vi "labview_data Writer Example.vi"() -> ()   [LabVIEW 2024]
uses:
  <vilib>/RTI DDS Toolkit/Types/RTI DDS Advanced Writer Configuration.ctl
  <vilib>/RTI DDS Toolkit/Library/LVDDS_library.lvlib
panel:
  in  "Sample":T1
  in  "Sample Type":T1
  in  "Advanced Writer Configuration":T2
  in  "error in (no error)":errorcluster
  in  "Stop Writing":bool
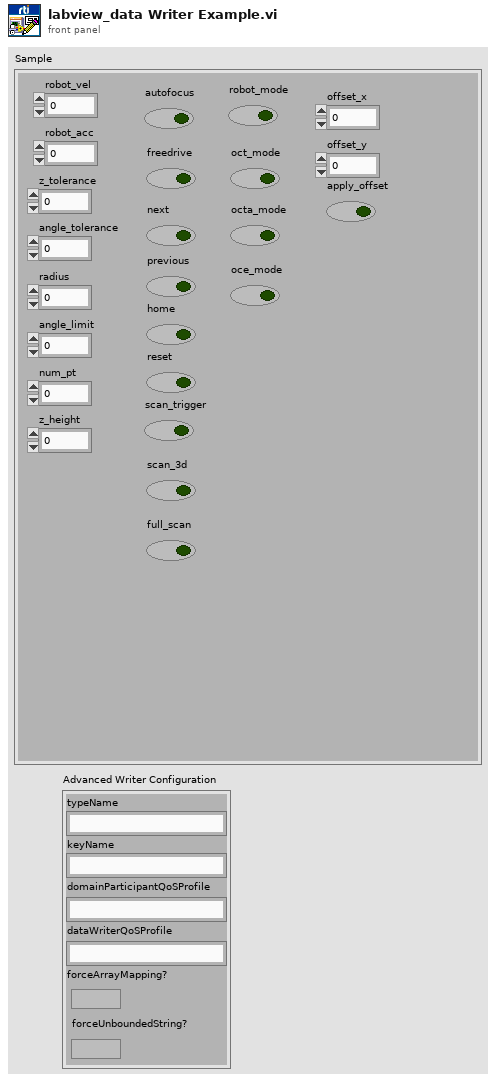
[diagram p1: front panel]
types:
  T1 = cluster{"robot_vel":dbl, "robot_acc":dbl, "z_tolerance":dbl, "angle_tolerance":dbl, "radius":dbl, "angle_limit":dbl, "num_pt":i32, "z_height":dbl, "autofocus":bool, "freedrive":bool, "next":bool, "previous":bool, "home":bool, "reset":bool, "scan_trigger":bool, "scan_3d":bool, "full_scan":bool, "robot_mode":bool, "oct_mode":bool, "octa_mode":bool, "oce_mode":bool, "offset_x":dbl, "offset_y":dbl, "apply_offset":bool}
  T2 = typedef "LVDDS_library.lvlib/RTI DDS Advanced Writer Configuration.ctl" = cluster{"typeName":string, "keyName":string, "domainParticipantQoSProfile":string, "dataWriterQoSProfile":string, "forceArrayMapping?":bool, "forceUnboundedString?":bool}
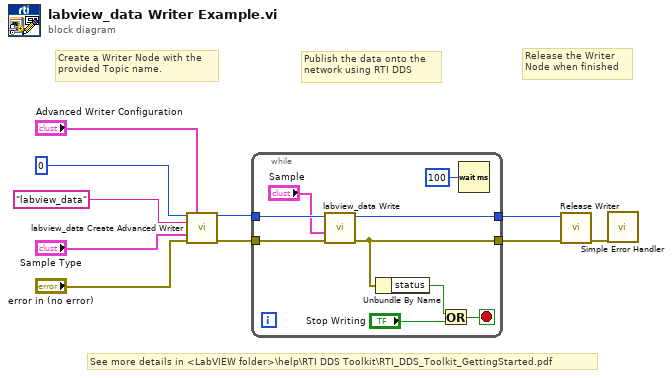
[diagram p0: block diagram]
diagram:
  # "See more details in <LabVIEW folder>\\help\\RTI DDS Toolkit\\RTI_DDS_Toolkit_GettingStarted.pdf"
  # "Release the Writer\nNode when finished"
  # "Publish the data onto the \nnetwork using RTI DDS"
  # "Create a Writer Node with the \nprovided Topic name."
  n1 = call "labview_data Create Advanced Writer.vi"("Domain Id"=u32 0, "Advanced Writer Configuration"="Advanced Writer Configuration", "Topic Name"="labview_data", "MyComplexType type"="Sample Type", "error in (no error)"="error in (no error)") -> ("DDS Object Ref"=w6:u64, "error out"=w7:errorcluster)  [unwired: 9 in]
  n2 = while "Main Loop" {
    tunnel: w6 -> [w19]
    tunnel: [w17] -> w10
    tunnel: w7 -> [w16]
    tunnel: [w14] -> w9
    stop <- w12 stop-if-true
    n3 = call "labview_data Write.vi"("error in (no error)"=w16, "MyComplexType"="Sample", "DDS Object Ref in"=w19) -> ("error out"=w14:errorcluster, "DDS Object Ref out"=w17:u64)  [unwired: 7 in]
    n4 = Unbundle By Name(w14) -> ("status"=w15:bool)
    n5 = Or(x=w15, y="Stop Writing") -> (x .or. y?=w12:bool)
    n6 = Wait (ms)(milliseconds to wait=u32 100 ("millisecond multiple")) -> ()  [unwired: 1 out]
  }
  n7 = call <vilib>:"Release Writer.vi"("error in (no error)"=w9, "DDS Object Ref"=w10) -> ("error out"=w8:errorcluster)  [unwired: 9 in]
  n8 = call <vilib>:"Simple Error Handler.vi"("error in (no error)"=w8) -> ()  [unwired: 4 in, 5 out]
